vi "API_ExecuteCommand.vi"(6 "Timeout (ms)":u32=10000, 7 "Wait (F)":bool=TRUE, 8 "error in (no error)":errorcluster, 10 "String":string, 11 "GIS Printer in":refnum<class "GIS Printer.lvclass">) -> (0 "error out":errorcluster, 1 "Aborted":bool, 2 "TimedOut":bool, 3 "GIS Printer out":refnum<class "GIS Printer.lvclass">)   [LabVIEW 2022 SP3, in "GIS Printer.lvclass"]
uses:
  GIS Printer.lvclass
  Typedefs/API Command Cluster.ctl
  Typedefs/API Command Enum.ctl
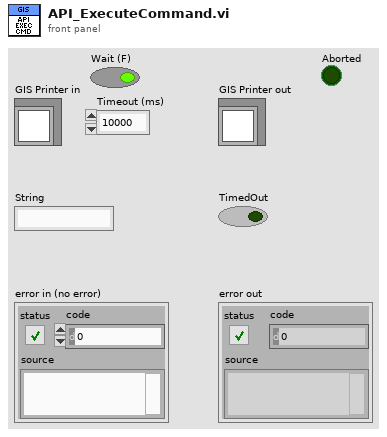
[diagram p1: front panel]
types:
  T1 = typedef "GIS Printer.lvclass/API Command Enum.ctl" = enum16{"Execute Printer Command", "Abort"}
  T2 = typedef "GIS Printer.lvclass/API Command Cluster.ctl" = cluster{"Command":T1, "Arguments":string}
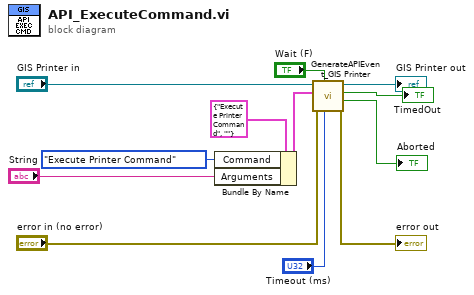
[diagram p0: block diagram]
diagram:
  n1 = Bundle By Name(cluster=T2 {"Command"=enum."Execute Printer Command", "Arguments"=""} ("API Command Cluster"), "Command"=API_Command_Enum."Execute Printer Command", "Arguments"="String") -> (w6:T2)
  n2 = call-dynamic "GenerateAPIEvent_GIS Printer.vi"("Timeout (ms)"="Timeout (ms)", "Wait (F)"="Wait (F)", "error in (no error)"="error in (no error)", "API Command Cluster"=w6, "GIS Printer in"="GIS Printer in") -> ("error out"=→"error out":errorcluster, "Aborted"=→"Aborted":bool, "TimedOut"=→"TimedOut":bool, "GIS Printer out"=→"GIS Printer out":refnum<class "GIS Printer.lvclass">)  [unwired: 3 in]
